vi "RSNRPZ Configure Averaging NS Ratio.vi"(7 "Upper Time Limit (4.0 s)":dbl=4.0 format="%.2p", 8 "error in (no error)":errorcluster, 9 "Maximum Noise Ratio (0.1 dB)":dbl=0.1 format="%.2p", 10 "Channel (1)":i32=1, 11 "VISA session":refnum<visa-resource-name> caption="VISA resource name") -> (0 "error out":errorcluster, 3 "dup VISA session":refnum<visa-resource-name> caption="VISA resource name")   [LabVIEW 2010]
doc: "This VI configures all parameters necessary for setting the noise ratio in the measurement result and automatic detection of filter bandwidth.\n\nRemote-control command(s):\nSENS:AVER:COUN:AUTO ON\nSENS:AVER:COUN:AUTO:TYPE NSR\nSENS:AVER:COUN:AUTO:NSR <value>\nSENS:AVER:COUN:AUTO:MTIM <value>\nSENS:AVER:TCON REP"
uses:
  rsnrpz_32.dll
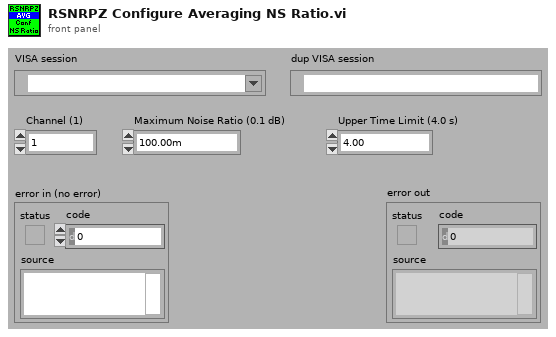
[diagram p1: front panel]
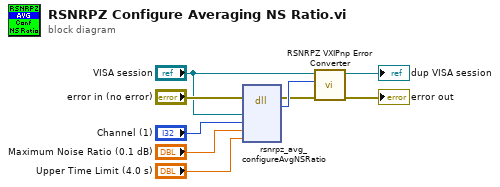
[diagram p0: block diagram]
diagram:
  n1 = dll-call lib="rsnrpz_32.dll" fn="rsnrpz_avg_configureAvgNSRatio"(error in="error in (no error)", "VISA Session"="VISA session", "Channel"="Channel (1)", "Maximum Noise Ratio"="Maximum Noise Ratio (0.1 dB)", "Upper Time Limit"="Upper Time Limit (4.0 s)") -> (error out=w5:errorcluster, "Status"=w9:i32)  [unwired: 6 in, 1 out]
  n2 = call <instrlib>:"RSNRPZ VXIPnp Error Converter.vi"("error in"=w5, "VXIPnp error code"=w9, "VISA session"="VISA session") -> ("error out"=→"error out":errorcluster, "dup VISA session"=→"dup VISA session":refnum<visa-resource-name>)  [unwired: 7 in]
